vi "Sync test.vi"() -> ()   [LabVIEW 2019]
uses:
  <vilib>/FPGAPlugInAG/sbRIO-9606/niLvFpga_Open_sbRIO-9606.vi
  <vilib>/rvi/interface/common/dynamic/niFpgaDynamicAddResources.vi
  <vilib>/FPGAPlugInAG/Dynamic/niLvFpga_Abort_Dynamic.vi
  <vilib>/FPGAPlugInAG/Dynamic/niLvFpga_Reset_Dynamic.vi
  <vilib>/Utility/error.llb/Error Cluster From Error Code.vi
  <vilib>/rvi/errors/niLvFpgaAdjustHostInterfaceError.vi
  <vilib>/FPGAPlugInAG/Dynamic/niLvFpga_Run_Dynamic.vi
  <vilib>/FPGAPlugInAG/Dynamic/niLvFpga_Close_Dynamic.vi
  <vilib>/rvi/interface/nirviOpenFPGA/nirviOpenFPGA.xnode
  FPGA Bitfiles/sbriotest_SecondFPGATarget_SecondBoardScope_yHmmvr9YX7w.lvbitx
  FPGA Bitfiles/sbriotest_MainFPGATarget_MainBoardScopeSy_ovSNDWeJdVk.lvbitx
  <vilib>/rvi/interface/nirviMethod/nirviMethod.xnode
  <vilib>/rvi/interface/nirviReadWriteControl/nirviReadWriteControl.xnode
  <vilib>/rvi/interface/nirviCloseFPGA/nirviCloseFPGA.xnode
  <vilib>/rvi/interface/Simulation/niFpgaSimulationCallBeginRW.vi
  NiFpgaLv.dll
panel:
  in  "Tab Control":enum32{"Scope Sync test", "Forced Clock Test"}(tab)
  in  "Single DIO/Bulk DIO":bool
  in  "Ring":u16(ring) items=["10 ticks", "50 ticks", "1 us", "1 ms", "100 ms", "1000 ms", "1 min"]
  in  "iter":u16
  in  "stop":bool
  # "Main Board:\nDIO63 - Sync(out)\nDIO48 - Scope(out)"
  # "Aux Board:\nDIO80 - Sync(in)\nDIO83 - Scope(out)"
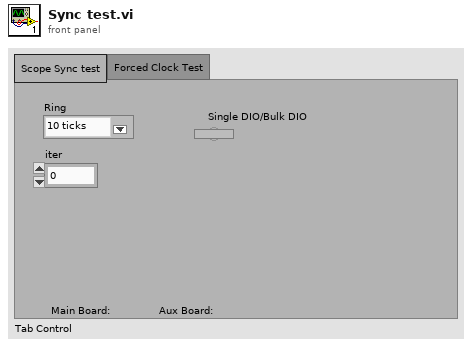
[diagram p1: front panel]
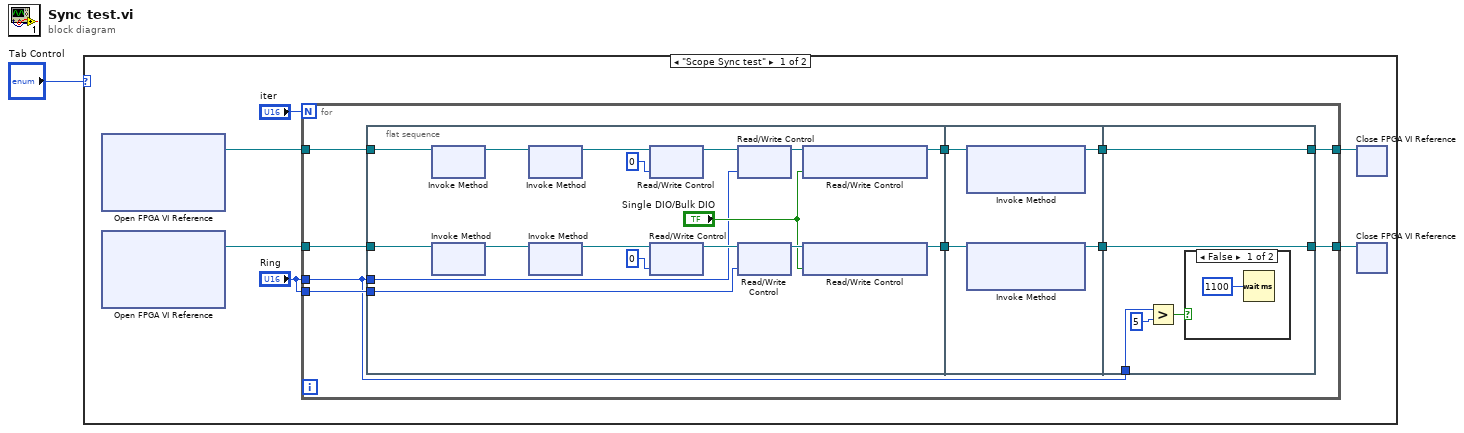
[diagram p0: block diagram]
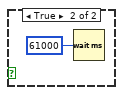
[diagram p2: hidden frame]
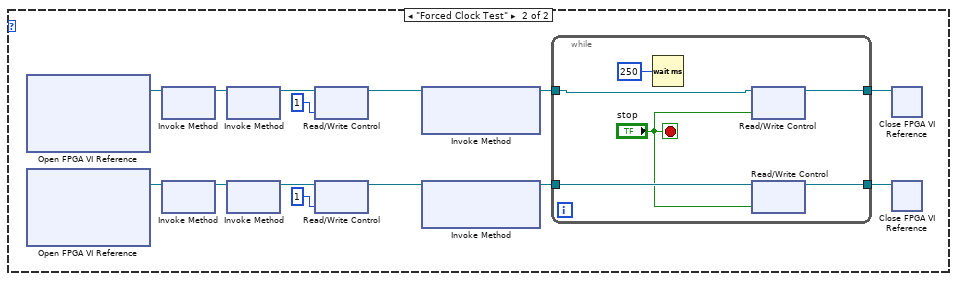
[diagram p3: hidden frame]
diagram:
  n1 = case shown="\"Scope Sync test\"" "Tab Control" {
    frame "Scope Sync test" {
      n2 = xnode "Open FPGA VI Reference"() -> ("FPGA VI Reference Out"=w5:refnum<k20>)  [unwired: 2 in, 1 out]
      n3 = xnode "Open FPGA VI Reference"() -> ("FPGA VI Reference Out"=w4:refnum<k20>)  [unwired: 2 in, 1 out]
      n4 = for {
        N: "iter" -> [_]
        tunnel: "Ring" -> [w17]
        tunnel: "Ring" -> [w8]
        tunnel: [w12] -> w3
        tunnel: [w11] -> w2
        tunnel: w5 -> [w16]
        tunnel: w4 -> [w15]
        n5 = flat-sequence {
          tunnel: w17 -> [w30]
          tunnel: w16 -> [w27]
          tunnel: w15 -> [w26]
          tunnel: w8 -> [w18]
          tunnel: [w25] -> w14
          tunnel: [w24] -> w13
          tunnel: w14 -> [w38]
          tunnel: w13 -> [w37]
          tunnel: [w36] -> w10
          tunnel: [w35] -> w9
          tunnel: [w42] -> w11
          tunnel: [w43] -> w12
          tunnel: w10 -> [w43]
          tunnel: w9 -> [w42]
          tunnel: w8 -> [w40]
          frame #0 {
            n6 = xnode "Invoke Method"("FPGA VI Reference In"=w27) -> ("FPGA VI Reference Out"=w29:refnum<k20>)  [unwired: 1 in, 1 out]
            n7 = xnode "Invoke Method"("FPGA VI Reference In"=w26) -> ("FPGA VI Reference Out"=w28:refnum<k20>)  [unwired: 1 in, 1 out]
            n8 = xnode "Invoke Method"("FPGA VI Reference In"=w29) -> ("FPGA VI Reference Out"=w32:refnum<k20>)  [unwired: 1 in, 1 out]
            n9 = xnode "Invoke Method"("FPGA VI Reference In"=w28) -> ("FPGA VI Reference Out"=w31:refnum<k20>)  [unwired: 1 in, 1 out]
            n10 = xnode "Read/Write Control"("FPGA VI Reference In"=w32, "Ring"=i16 0) -> ("FPGA VI Reference Out"=w22:refnum<k20>)  [unwired: 1 in, 1 out]
            n11 = xnode "Read/Write Control"("FPGA VI Reference In"=w31, "Ring"=i16 0) -> ("FPGA VI Reference Out"=w21:refnum<k20>)  [unwired: 1 in, 1 out]
            n12 = xnode "Read/Write Control"("FPGA VI Reference In"=w22, "Delay"=w18) -> ("FPGA VI Reference Out"=w33:refnum<k20>)  [unwired: 1 in, 1 out]
            n13 = xnode "Read/Write Control"("FPGA VI Reference In"=w21, "Delay"=w30) -> ("FPGA VI Reference Out"=w34:refnum<k20>)  [unwired: 1 in, 1 out]
            n14 = xnode "Read/Write Control"("FPGA VI Reference In"=w33, "Single DIO/Bulk DIO"="Single DIO/Bulk DIO") -> ("FPGA VI Reference Out"=w25:refnum<k20>)  [unwired: 1 in, 1 out]
            n15 = xnode "Read/Write Control"("FPGA VI Reference In"=w34, "Single DIO/Bulk DIO"="Single DIO/Bulk DIO") -> ("FPGA VI Reference Out"=w24:refnum<k20>)  [unwired: 1 in, 1 out]
          }
          frame #1 {
            n16 = xnode "Invoke Method"("FPGA VI Reference In"=w38) -> ("FPGA VI Reference Out"=w36:refnum<k20>)  [unwired: 2 in, 1 out]
            n17 = xnode "Invoke Method"("FPGA VI Reference In"=w37) -> ("FPGA VI Reference Out"=w35:refnum<k20>)  [unwired: 2 in, 1 out]
          }
          frame #2 {
            n18 = Greater?(x=w40, y=u8 5) -> (0:w39:bool)
            n19 = case shown="False" w39 {
              frame False {
                n20 = Wait (ms)(milliseconds to wait=u32 1100) -> ()  [unwired: 1 out]
              }
              frame True {
                n21 = Wait (ms)(milliseconds to wait=u32 61000) -> ()  [unwired: 1 out]
              }
            }
          }
        }
      }
      n22 = xnode "Close FPGA VI Reference"("FPGA VI Reference In"=w3) -> ()  [unwired: 1 in, 1 out]
      n23 = xnode "Close FPGA VI Reference"("FPGA VI Reference In"=w2) -> ()  [unwired: 1 in, 1 out]
    }
    frame "Forced Clock Test" {
      n24 = xnode "Open FPGA VI Reference"() -> ("FPGA VI Reference Out"=w51:refnum<k20>)  [unwired: 2 in, 1 out]
      n25 = xnode "Open FPGA VI Reference"() -> ("FPGA VI Reference Out"=w50:refnum<k20>)  [unwired: 2 in, 1 out]
      n26 = xnode "Invoke Method"("FPGA VI Reference In"=w51) -> ("FPGA VI Reference Out"=w56:refnum<k20>)  [unwired: 1 in, 1 out]
      n27 = xnode "Invoke Method"("FPGA VI Reference In"=w50) -> ("FPGA VI Reference Out"=w57:refnum<k20>)  [unwired: 1 in, 1 out]
      n28 = xnode "Invoke Method"("FPGA VI Reference In"=w56) -> ("FPGA VI Reference Out"=w54:refnum<k20>)  [unwired: 1 in, 1 out]
      n29 = xnode "Invoke Method"("FPGA VI Reference In"=w57) -> ("FPGA VI Reference Out"=w55:refnum<k20>)  [unwired: 1 in, 1 out]
      n30 = xnode "Read/Write Control"("FPGA VI Reference In"=w54, "Ring"=i16 1) -> ("FPGA VI Reference Out"=w58:refnum<k20>)  [unwired: 1 in, 1 out]
      n31 = xnode "Read/Write Control"("FPGA VI Reference In"=w55, "Ring"=i16 1) -> ("FPGA VI Reference Out"=w59:refnum<k20>)  [unwired: 1 in, 1 out]
      n32 = xnode "Invoke Method"("FPGA VI Reference In"=w58) -> ("FPGA VI Reference Out"=w49:refnum<k20>)  [unwired: 2 in, 1 out]
      n33 = xnode "Invoke Method"("FPGA VI Reference In"=w59) -> ("FPGA VI Reference Out"=w48:refnum<k20>)  [unwired: 2 in, 1 out]
      n34 = while {
        tunnel: w48 -> [w64]
        tunnel: w49 -> [w65]
        tunnel: [w61] -> w47
        tunnel: [w60] -> w46
        stop <- "stop" stop-if-true
        n35 = Wait (ms)(milliseconds to wait=u32 250) -> ()  [unwired: 1 out]
        n36 = xnode "Read/Write Control"("FPGA VI Reference In"=w65, "stop"="stop") -> ("FPGA VI Reference Out"=w60:refnum<k20>)  [unwired: 1 in, 1 out]
        n37 = xnode "Read/Write Control"("FPGA VI Reference In"=w64, "stop"="stop") -> ("FPGA VI Reference Out"=w61:refnum<k20>)  [unwired: 1 in, 1 out]
      }
      n38 = xnode "Close FPGA VI Reference"("FPGA VI Reference In"=w46) -> ()  [unwired: 1 in, 1 out]
      n39 = xnode "Close FPGA VI Reference"("FPGA VI Reference In"=w47) -> ()  [unwired: 1 in, 1 out]
    }
  }
